vi "DB_EscribeTablaMediciones.vi"(8 "error in (no error)":errorcluster, 10 "Equipo_Medicion in":T1={"ID_EQUIPO"=0, "IP_EQUIPO"="", "NOMBRE_EQUIPO"="", "ESTADO_EQUIPO"="", "DESCRIPCION"="", "ID_MEDICION"=0, "ESTADO_MEDICION"="", "TIEMPO_MEDICION"="12-02-2019 18:41"}, 11 "db in":T2) -> (0 "error out":errorcluster, 3 "db out":T2)   [LabVIEW 2018]
uses:
  <vilib>/addons/database/Connection.llb/Conn ObjectReference.ctl
  Controls/Equipos_Medicion_cluster.ctl
  <vilib>/addons/database/Connection.llb/Conn Execute.vi
  <vilib>/addons/database/Recordset.llb/Rec Destroy - Connection.vi
  <vilib>/addons/database/NI_Database_API.lvlib
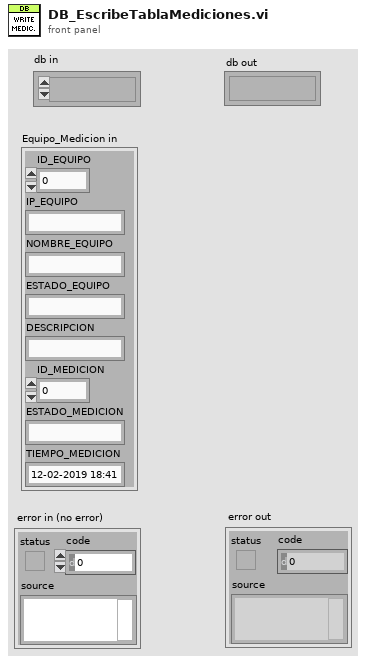
[diagram p1: front panel]
types:
  T1 = typedef "Equipos_Medicion_cluster.ctl" = cluster{"ID_EQUIPO":i32, "IP_EQUIPO":string, "NOMBRE_EQUIPO":string, "ESTADO_EQUIPO":string, "DESCRIPCION":string, "ID_MEDICION":i32, "ESTADO_MEDICION":string, "TIEMPO_MEDICION":string}
  T2 = typedef "NI_Database_API.lvlib/Conn ObjectReference.ctl" = refnum<k1>
  T3 = typedef "NI_Database_API.lvlib/Rec ObjectReference.ctl" = refnum<k1>
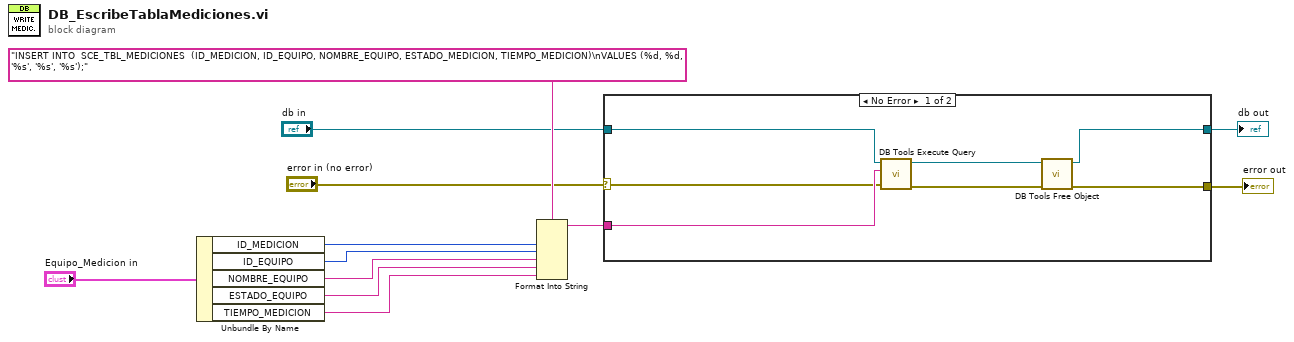
[diagram p0: block diagram]
diagram:
  n1 = Unbundle By Name("Equipo_Medicion in") -> ("ID_MEDICION"=w2:i32, "ID_EQUIPO"=w1:i32, "NOMBRE_EQUIPO"=w8:string, "ESTADO_EQUIPO"=w7:string, "TIEMPO_MEDICION"=w6:string)
  n2 = Format Into String(format string="INSERT INTO  SCE_TBL_MEDICIONES  (ID_MEDICION, ID_EQUIPO, NOMBRE_EQUIPO, ESTADO_MEDICION, TIEMPO_MEDICION)\nVALUES (%d, %d, '%s', '%s', '%s');" ("SQL"), w2, w1, w8, w7, w6) -> (resulting string=w12:string)  [unwired: 2 in, 1 out]
  n3 = case shown="No Error" "error in (no error)" {
    selector: "error in (no error)" -> [w17 w21]
    tunnel: w12 -> [w18 _]
    tunnel: [w15 w21] -> w10
    tunnel: "db in" -> [w16 w20]
    tunnel: [w13 w20] -> w4
    frame No Error {
      n4 = call-poly <vilib>:"DB Tools Execute Query.vi"("error in (no error)"=w17, "SQL query"=w18, "connection reference"=w16) -> ("error out"=w19:errorcluster, "recordset reference"=w14:T3)  [unwired: 5 in]
      n5 = call-poly <vilib>:"DB Tools Free Object.vi"("error in (no error)"=w19, "recordset reference"=w14) -> ("error out"=w15:errorcluster, "connection reference"=w13:T2)  [unwired: 8 in]
    }
    frame Error {
    }
  }
  "error out" <- w10
  "db out" <- w4
